vi "EstimateGamePiece.vi"(1 "Acceptable GamePiece Radius (in)":dbl=5.0 format="%#_13g", 2 "Robot X (in) [t0]":dbl, 3 "Robot Y (in) [t0]":dbl, 7 "GamePiece Type [t-?]":enum16{"None", "Cube", "Cone"}(ring), 9 "GamePiece Confidence [t-?]":dbl, 11 "GamePiece Timestamp (ms)":u32, 12 "GamePiece Y (in) [t-?]":dbl, 13 "GamePiece X (in) [t-?]":dbl, 14 "GamePiece Valid [t-?]":bool, 15 "GamePiece Range (in) [t-?]":dbl) -> (8 "Sorted GamePiece Instances":T1(array[cluster]))   [LabVIEW 2020]
doc: "Searches through all recent game piece observations, and assigns each observation to a cluster. For each cluster, define a unique game piece instance and rank them according to a fitness score."
uses:
  GlobalArm.vi
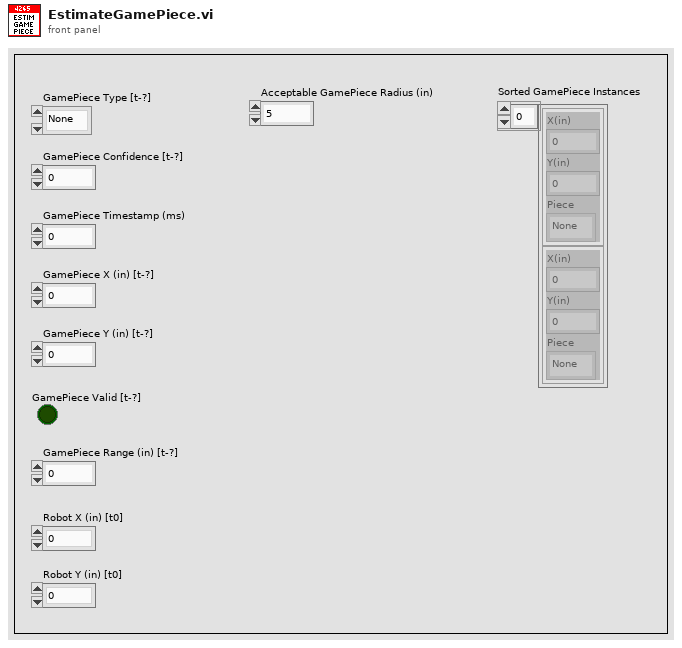
[diagram p1: front panel]
types:
  T1 = cluster{"X(in)":dbl, "Y(in)":dbl, "Piece":enum16{"None", "Cube", "Cone"}}[]
  T2 = cluster{"X":dbl, "Y":dbl, "Vision Timestamp (ms)":u32, "Confidence":dbl, "Range":dbl, "Piece":enum16{"None", "Cube", "Cone"}}
  T3 = cluster{"X":dbl, "Y":dbl, "Vision Timestamp (ms)":u32, "Confidence":dbl, "Range":dbl, "Piece":enum16{"None", "Cube", "Cone"}}[]
  T4 = cluster{"X(in)":dbl, "Y(in)":dbl, "Count":i32, "Timestamp(ms)":u32, "Piece":enum16{"None", "Cube", "Cone"}}
  T5 = cluster{"X(in)":dbl, "Y(in)":dbl, "Piece":enum16{"None", "Cube", "Cone"}}
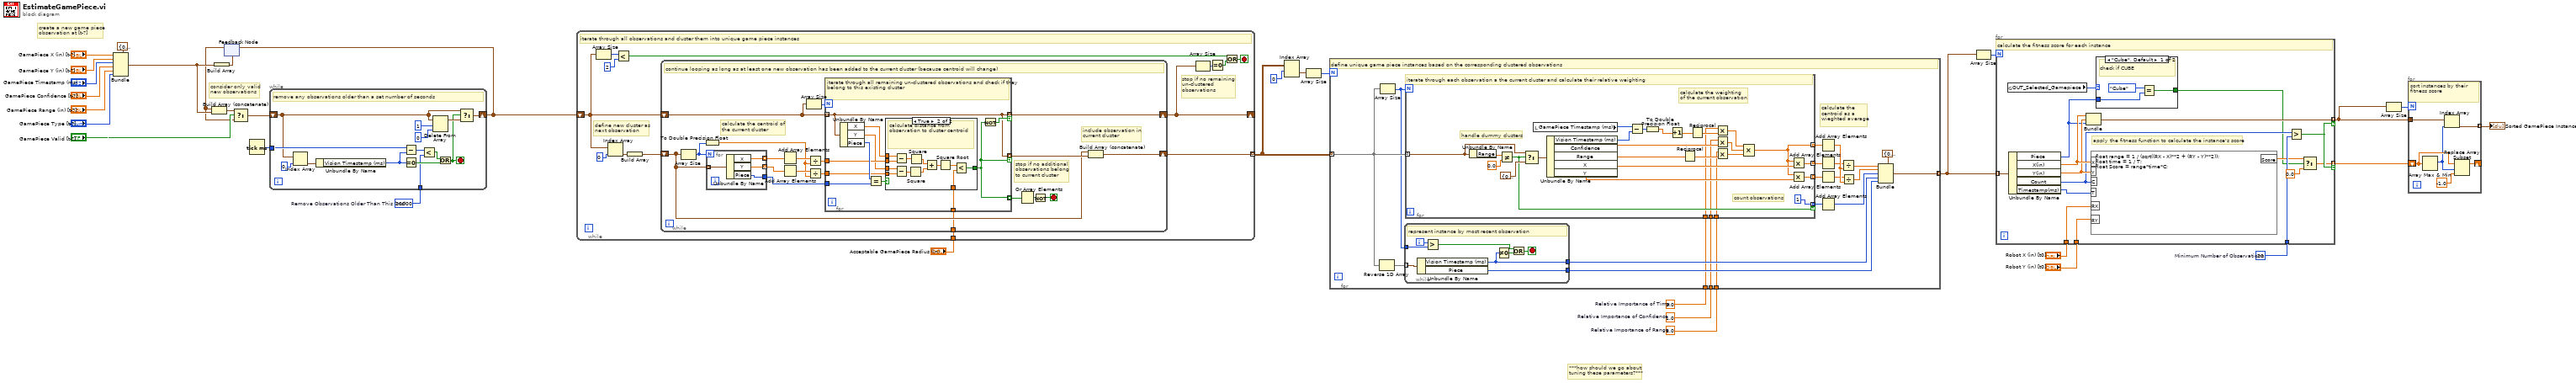
[diagram p0: block diagram]
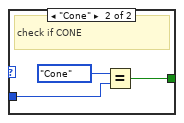
[diagram p2: hidden frame]
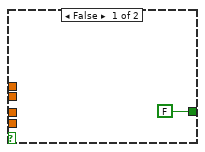
[diagram p3: hidden frame]
diagram:
  w3 = 20  # Minimum Number of Observations
  w4 = 1.0  # Relative Importance of Range
  w5 = 1.0  # Relative Importance of Confidence
  w6 = 1.0  # Relative Importance of Time
  w7 = u32 20000  # Remove Observations Older Than This (ms)
  # "***how should we go about\ntuning these parameters?***"
  # "consider only valid\nnew observations"
  # "create a new game piece\nobservation at [t-?]"
  n1 = Bundle(cluster=T2 {"X"=0.0, "Y"=0.0, "Vision Timestamp (ms)"=0, "Confidence"=0.0, "Range"=1.0, "Piece"=enum."None"} ("Cluster"), "X"="GamePiece X (in) [t-?]", "Y"="GamePiece Y (in) [t-?]", "Vision Timestamp (ms)"="GamePiece Timestamp (ms)", "Confidence"="GamePiece Confidence [t-?]", "Range"="GamePiece Range (in) [t-?]", "Piece"="GamePiece Type [t-?]") -> (w24:T2)
  n2 = Build Array(w24) -> (w23:T3)
  n3 = feedback #1(w23) -> (w12:T3)
  n4 = Build Array (concatenate)(w12, w24) -> (w14:T3)
  n5 = Select(t=w14, s="GamePiece Valid [t-?]", f=w12) -> (s? t:f=w15:T3)
  n6 = Tick Count (ms)() -> (millisecond timer value=w9:u32)
  n7 = while {
    tunnel: w9 -> [w45]
    shift-right: [w39] -> w11
    shift-left: w15 -> [w41]
    tunnel: w7 -> [w34]
    stop <- w35 stop-if-true
    # "remove any observations older than a set number of seconds"
    n8 = Index Array(array=w41, index=0) -> (element=w46:T2)
    n9 = Unbundle By Name(w46) -> ("Vision Timestamp (ms)"=w38:u32)
    n10 = Subtract(x=w45, y=w38) -> (x-y=w44:u32)
    n11 = Equal To 0?(x=w38) -> (x = 0?=w37:bool)
    n12 = Less?(x=w44, y=w34) -> (x < y?=w36:bool)
    n13 = Delete From Array(array=w41, length=1, index=0) -> (array with subset deleted=w40:T3)  [unwired: 1 out]
    n14 = Or(x=w36, y=w37) -> (x .or. y?=w35:bool)
    n15 = Select(t=w41, s=w35, f=w40) -> (s? t:f=w39:T3)
  }
  n16 = feedback-in #1(w11) -> ()
  n17 = while {
    shift-right: [w51] -> _
    shift-left: w11 -> [w55]
    tunnel: [w52] -> w21 mode=indexing
    tunnel: "Acceptable GamePiece Radius (in)" -> [w50]
    stop <- w57 stop-if-true
    # "define new cluster as\nnext observation"
    # "stop if no remaining\nun-clustered\nobservations"
    # "iterate through all observations and cluster them into unique game piece instances"
    n18 = Array Size(array=w55) -> (size(s)=w59:i32)
    n19 = Index Array(array=w55, index=0) -> (element=w54:T2)
    n20 = Less?(x=w59, y=2) -> (x < y?=w49:bool)
    n21 = Build Array(w54) -> (w53:T3)
    n22 = while {
      shift-right: [w70] -> w51
      shift-left: w55 -> [w63]
      shift-right: [w67] -> w52
      shift-left: w53 -> [w68]
      tunnel: w50 -> [w61]
      stop <- w64 stop-if-true
      # "include observation in\ncurrent cluster"
      # "stop if no additional\nobservations belong\nto current cluster"
      # "calculate the centroid of\nthe current cluster"
      # "continue looping as long as at least one new observation has been added to the current cluster (because centroid will change)"
      n23 = Array Size(array=w68) -> (size(s)=w74:i32)
      n24 = To Double Precision Float(number=w74) -> (double precision float=w71:dbl)
      n25 = for {
        N: w74 -> [_]
        tunnel: w68 -> [w83] mode=indexing
        tunnel: [w82] -> w79 mode=indexing
        tunnel: [w81] -> w78 mode=indexing
        tunnel: [w80] -> w77
        n26 = Unbundle By Name(w83) -> ("X"=w82:dbl, "Y"=w81:dbl, "Piece"=w80:enum16{"None", "Cube", "Cone"})
      }
      n27 = Add Array Elements(numeric array=w79) -> (sum=w75:dbl)
      n28 = Add Array Elements(numeric array=w78) -> (sum=w73:dbl)
      n29 = Array Size(array=w63) -> (size(s)=w62:i32)
      n30 = Divide(x=w75, y=w71) -> (x/y=w76:dbl)
      n31 = Divide(x=w73, y=w71) -> (x/y=w72:dbl)
      n32 = for {
        N: w62 -> [_]
        tunnel: w63 -> [w93] mode=indexing
        tunnel: [w93] -> w69 mode=indexing if=w88
        tunnel: [w93] -> w70 mode=indexing if=w94
        tunnel: w76 -> [w86]
        tunnel: w72 -> [w85]
        tunnel: w77 -> [w91]
        tunnel: [w88] -> w66 mode=indexing
        tunnel: w61 -> [w89]
        # "iterate through all remaining un-clustered observations and check if they belong to this existing cluster"
        n33 = Unbundle By Name(w93) -> ("X"=w87:dbl, "Y"=w84:dbl, "Piece"=w92:enum16{"None", "Cube", "Cone"})
        n34 = Equal?(x=w92, y=w91) -> (x = y?=w90:bool)
        n35 = case shown="True" w90 {
          tunnel: w87 -> [_ w101]
          tunnel: w86 -> [_ w100]
          tunnel: w84 -> [_ w99]
          tunnel: w85 -> [_ w98]
          tunnel: [FALSE w97] -> w88
          tunnel: w89 -> [_ w96]
          frame False {
          }
          frame True {
            # "calculate distance from observation to cluster centroid"
            n36 = Subtract(x=w101, y=w100) -> (x-y=w107:dbl)
            n37 = Subtract(x=w99, y=w98) -> (x-y=w106:dbl)
            n38 = Square(x=w106) -> (x^2=w104:dbl)
            n39 = Square(x=w107) -> (x^2=w105:dbl)
            n40 = Add(x=w105, y=w104) -> (x+y=w103:dbl)
            n41 = Square Root(x=w103) -> (sqrt(x)=w102:dbl)
            n42 = Less?(x=w102, y=w96) -> (x < y?=w97:bool)
          }
        }
        n43 = Not(x=w88) -> (.not. x?=w94:bool)
      }
      n44 = Or Array Elements(Boolean array=w66) -> (logical OR=w65:bool)
      n45 = Not(x=w65) -> (.not. x?=w64:bool)
      n46 = Build Array (concatenate)(w68, w69) -> (w67:T3)
    }
    n47 = Array Size(array=w51) -> (size(s)=w60:i32)
    n48 = Equal To 0?(x=w60) -> (x = 0?=w48:bool)
    n49 = Or(x=w49, y=w48) -> (x .or. y?=w57:bool)
  }
  n50 = Index Array(array=w21, index (row)=0) -> (element=w32:T3)  [unwired: 1 in]
  n51 = Array Size(array=w32) -> (size(s)=w33:i32)
  n52 = for {
    N: w33 -> [_]
    tunnel: w21 -> [w112] mode=indexing
    tunnel: [w123] -> w29 mode=indexing
    tunnel: w6 -> [w110]
    tunnel: w5 -> [w109]
    tunnel: w4 -> [w108]
    # "calculate the \ncentroid as a\nwieghted average"
    # "define unique game piece instances based on the corresponding clustered observations"
    n53 = Reverse 1D Array(array=w112) -> (reversed array=w116:T3)
    n54 = Array Size(array=w112) -> (size(s)=w111:i32)
    n55 = while {
      tunnel: [w134] -> w125
      tunnel: w116 -> [w135] mode=indexing
      tunnel: [w133] -> w113
      tunnel: w111 -> [w131]
      i -> [w132]
      stop <- w130 stop-if-true
      # "represent instance by most recent observation"
      n56 = Unbundle By Name(w135) -> ("Vision Timestamp (ms)"=w134:u32, "Piece"=w133:enum16{"None", "Cube", "Cone"})
      n57 = Greater?(x=w132, y=w131) -> (0:w129:bool)
      n58 = Not Equal To 0?(x=w134) -> (x != 0?=w128:bool)
      n59 = Or(x=w129, y=w128) -> (x .or. y?=w130:bool)
    }
    n60 = for {
      N: w111 -> [_]
      tunnel: w112 -> [w146] mode=indexing
      tunnel: [w138] -> w122 mode=indexing
      tunnel: [w152] -> w120 mode=indexing
      tunnel: [w143] -> w118 mode=indexing
      tunnel: [1] -> w115 mode=indexing if=w142
      tunnel: w110 -> [w141]
      tunnel: w109 -> [w140]
      tunnel: w108 -> [w139]
      # "calculate the weighting\nof the current observation"
      # "count observations"
      # "handle dummy clusters"
      # "iterate through each observation a the current cluster and calculate their relative weighting"
      n61 = Unbundle By Name(w146) -> ("Range"=w149:dbl)
      n62 = Not Equal?(x=w149, y=0.0) -> (x != y?=w142:bool)
      n63 = Select(t=w146, s=w142, f=T2 {"X"=0.0, "Y"=0.0, "Vision Timestamp (ms)"=1, "Confidence"=0.0, "Range"=1.0, "Piece"=enum."None"} ("Cluster")) -> (s? t:f=w145:T2)
      n64 = local read "GamePiece Timestamp (ms)"() -> (w161:u32)
      n65 = Unbundle By Name(w145) -> ("Vision Timestamp (ms)"=w162:u32, "Confidence"=w159:dbl, "Range"=w151:dbl, "X"=w156:dbl, "Y"=w155:dbl)
      n66 = Subtract(x=w161, y=w162) -> (x-y=w154:u32)
      n67 = To Double Precision Float(number=w154) -> (double precision float=w136:dbl)
      n68 = Increment(x=w136) -> (x+1=w137:dbl)
      n69 = Reciprocal(x=w151) -> (1/x=w153:dbl)
      n70 = Reciprocal(x=w137) -> (1/x=w160:dbl)
      n71 = Multiply(x=w141, y=w160) -> (x*y=w150:dbl)
      n72 = Multiply(x=w140, y=w159) -> (x*y=w158:dbl)
      n73 = Multiply(x=w139, y=w153) -> (x*y=w157:dbl)
      n74 = Compound Arithmetic op=MULTIPLY(w150, w158, w157) -> (w138:dbl)
      n75 = Multiply(x=w138, y=w156) -> (x*y=w143:dbl)
      n76 = Multiply(x=w138, y=w155) -> (x*y=w152:dbl)
    }
    n77 = Add Array Elements(numeric array=w122) -> (sum=w121:dbl)
    n78 = Add Array Elements(numeric array=w118) -> (sum=w117:dbl)
    n79 = Add Array Elements(numeric array=w120) -> (sum=w119:dbl)
    n80 = Add Array Elements(numeric array=w115) -> (sum=w114:i32)
    n81 = Divide(x=w117, y=w121) -> (x/y=w127:dbl)
    n82 = Divide(x=w119, y=w121) -> (x/y=w126:dbl)
    n83 = Bundle(cluster=T4 {"X(in)"=0.0, "Y(in)"=0.0, "Count"=0, "Timestamp(ms)"=0, "Piece"=enum."None"}, "X(in)"=w127, "Y(in)"=w126, "Count"=w114, "Timestamp(ms)"=w125, "Piece"=w113) -> (w123:T4)
  }
  n84 = Array Size(array=w29) -> (size(s)=w31:i32)
  n85 = for {
    N: w31 -> [_]
    tunnel: w29 -> [w178] mode=indexing
    tunnel: "Robot X (in) [t0]" -> [w173]
    tunnel: "Robot Y (in) [t0]" -> [w172]
    tunnel: [w164] -> w27 mode=indexing if=w167
    tunnel: [w177] -> w26 mode=indexing if=w167
    tunnel: w3 -> [w170]
    # "apply the fitness function to calculate the instance's score"
    # "calculate the fitness score for each instance"
    n86 = global read "GlobalArm.vi" "OUT_Selected_Gamepiece"() -> (w168:enum16{"Cube", "Cone"})
    n87 = Unbundle By Name(w178) -> ("Piece"=w169:enum16{"None", "Cube", "Cone"}, "X(in)"=w176:dbl, "Y(in)"=w175:dbl, "Count"=w171:i32, "Timestamp(ms)"=w174:u32)
    n88 = Bundle("X(in)"=w176, "Y(in)"=w175, "Piece"=w169) -> (w177:T5)  [unwired: 1 in]
    n89 = formula code="float range = 1 / (sqrt((RX - X)**2 + (RY - Y)**2));\nfloat time = 1 / T;\nfloat Score = range*time*C;"("X"=w176, "Y"=w175, "C"=w171, "T"=w174, "RY"=w172, "RX"=w173) -> ("Score"=w166:dbl)
    n90 = case shown="\"Cube\", Default" w168 {
      tunnel: w169 -> [w181 w182]
      tunnel: [w180 w183] -> w163
      frame "Cube", Default {
        # "check if CUBE"
        n91 = Equal?(x=enum16{"None", "Cube", "Cone"}."Cube", y=w181) -> (x = y?=w180:bool)
      }
      frame "Cone" {
        # "check if CONE"
        n92 = Equal?(x=enum16{"None", "Cube", "Cone"}."Cone", y=w182) -> (x = y?=w183:bool)
      }
    }
    n93 = Greater?(x=w171, y=w170) -> (0:w167:bool)
    n94 = Select(t=w166, s=w163, f=0.0) -> (s? t:f=w164:dbl)
  }
  n95 = Array Size(array=w26) -> (size(s)=w28:i32)
  n96 = for {
    N: w28 -> [_]
    tunnel: w26 -> [w190]
    shift-right: [w188] -> _
    shift-left: w27 -> [w187]
    tunnel: [w189] -> w22 mode=indexing
    # "sort instances by their fitness score"
    n97 = Array Max & Min(array=w187) -> (max index (indices)=w185:i32)  [unwired: 3 out]
    n98 = Index Array(array=w190, index=w185) -> (element=w189:T5)
    n99 = Replace Array Subset(array=w187, new element=-1.0 ("new element/subarray"), index=w185) -> (w188:dbl[])
  }
  "Sorted GamePiece Instances" <- w22
